vi "full adder (SubVI).vi"(2 "b":bool, 3 "c":bool, 4 "a":bool) -> (0 "sum":bool, 1 "carry":bool)   [LabVIEW 2012]
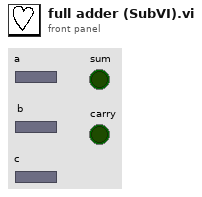
[diagram p1: front panel]
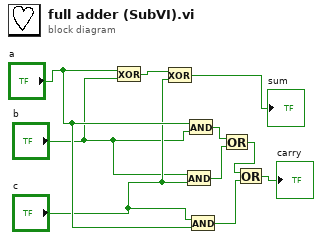
[diagram p0: block diagram]
diagram:
  n1 = Exclusive Or(1:"b", 2:"a") -> (0:w1:bool)
  n2 = Exclusive Or(1:"c", 2:w1) -> (0:→"sum":bool)
  n3 = And(x="b", y="c") -> (x .and. y?=w7:bool)
  n4 = And(x="a", y="b") -> (x .and. y?=w6:bool)
  n5 = And(x="c", y="a") -> (x .and. y?=w9:bool)
  n6 = Or(x=w6, y=w7) -> (x .or. y?=w8:bool)
  n7 = Or(x=w8, y=w9) -> (x .or. y?=→"carry":bool)
